vi "Load all Mesurements classes.vi"(8 "Error In":errorcluster) -> (0 "Error Out":errorcluster, 2 "Measurement classes":refnum<class "Measurement.lvclass">[](array[class]), 3 "Measurement names":string[](array[string]))   [LabVIEW 2020, in "Test Framework.lvclass"]
uses:
  Test Framework.lvclass
  Measurements/Measurement.lvclass
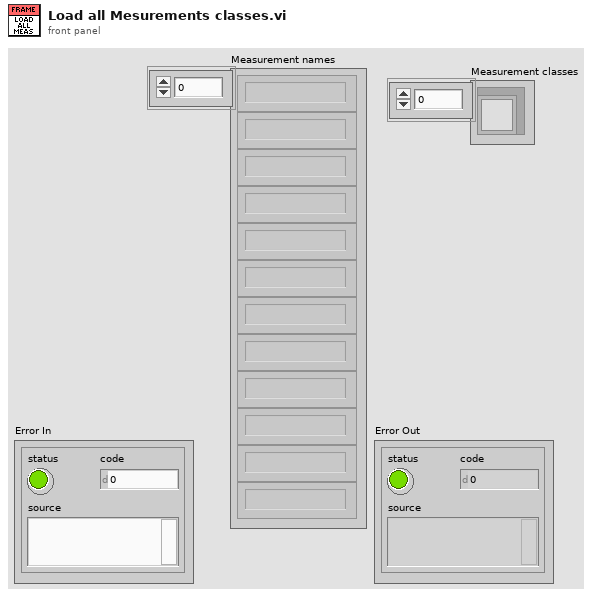
[diagram p1: front panel]
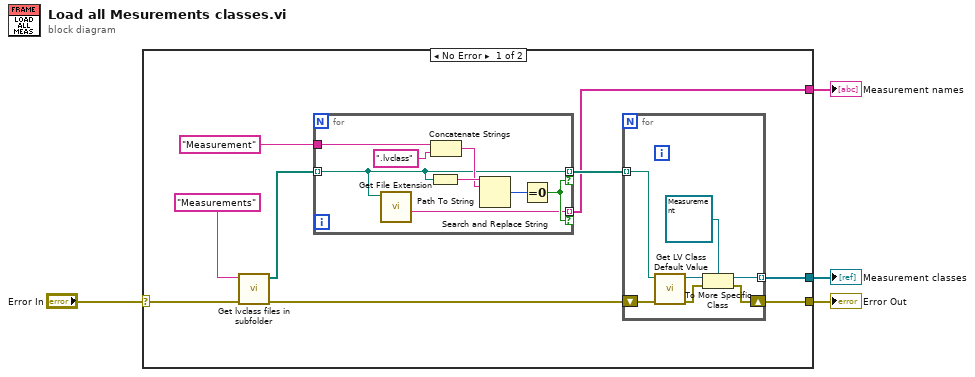
[diagram p0: block diagram]
diagram:
  n1 = case shown="No Error" "Error In" {
    selector: "Error In" -> [w13 w29]
    tunnel: [w8 _] -> w1
    tunnel: [w7 w29] -> w3
    tunnel: [w6 _] -> w2
    frame No Error {
      n2 = call "Get lvclass files in subfolder.vi"("Error In"=w13, "Sub Folder"="Measurements") -> ("Error Out"=w9:errorcluster, "Found lvclass files"=w11:path[])  [unwired: 8 in]
      n3 = for {
        tunnel: w11 -> [w22] mode=indexing
        tunnel: "Measurement" ("Sub Folder") -> [w26]
        tunnel: [w22] -> w10 mode=indexing if=w23
        tunnel: [w21] -> w6 mode=indexing if=w23
        n4 = call <vilib>:"Get File Extension.vi"("file"=w22) -> ("filename without extension"=w21:string)  [unwired: 6 in, 4 out]
        n5 = Path To String(path=w22) -> (string=w28:string)
        n6 = Concatenate Strings(w26, ".lvclass" ("string")) -> (w27:string)
        n7 = Search and Replace String(input string=w28, search string=w27) -> (number of replacements=w24:i32)  [unwired: 6 in, 3 out]
        n8 = Equal To 0?(x=w24) -> (x = 0?=w23:bool)
      }
      n9 = for {
        tunnel: w10 -> [w19] mode=indexing
        shift-right: [w16] -> w7
        shift-left: w9 -> [w20]
        tunnel: [w14] -> w8 mode=indexing
        n10 = call <vilib>:"Get LV Class Default Value.vi"("error in (no error)"=w20, "class path"=w19) -> ("error out"=w17:errorcluster, "object"=w18:refnum<class>)  [unwired: 8 in]
        n11 = To More Specific Class(target class=refnum<class "Measurement.lvclass"> refnum ("Measurements.lvclass"), reference=w18, error in=w17) -> (specific class reference=w14:refnum<class "Measurement.lvclass">, error out=w16:errorcluster)
      }
    }
    frame Error {
    }
  }
  "Error Out" <- w3
  "Measurement names" <- w2
  "Measurement classes" <- w1
